vi "symmetry property.vi"() -> ()   [LabVIEW 2014]
panel:
  out "Waveform Chart":dbl[][](graph)
  out "Waveform Chart 2":dbl[][](graph)
  out "OUTPUT 2":cdb[](array[numeric])
  in  "N 2":dbl
  in  "N":dbl
  in  "stop 2":bool
  out "OUTPUT-1":cdb[](array[numeric])
  in  "stop":bool
  # "SYMMETRY PROPERTY-1"
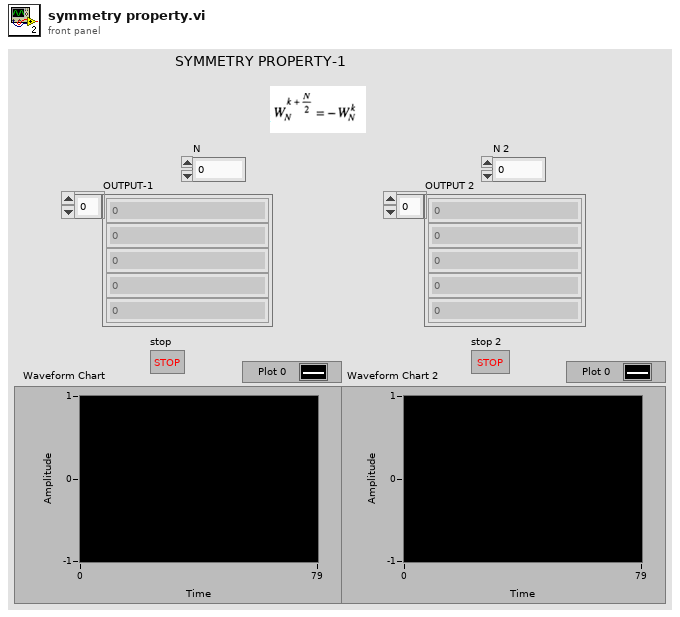
[diagram p1: front panel]
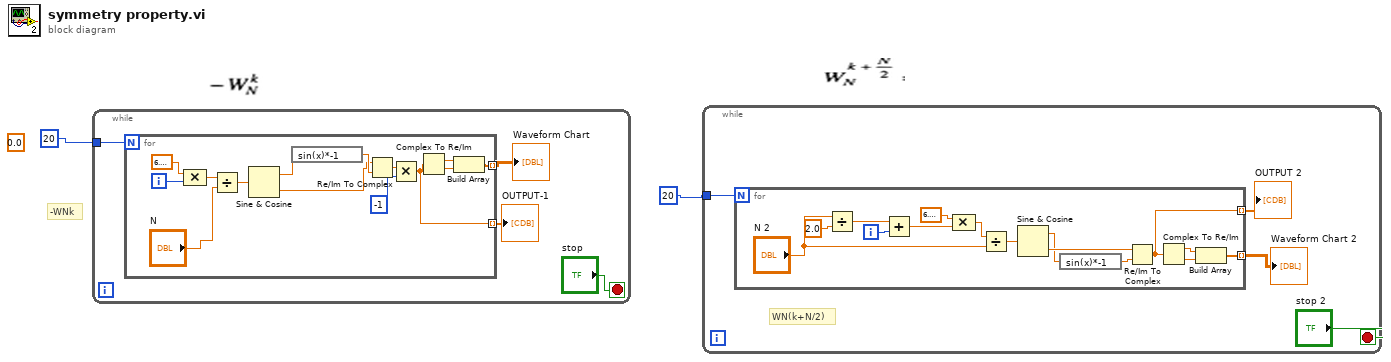
[diagram p0: block diagram]
diagram:
  (unwired) 0.0 ("Numeric")
  # "-WNk"
  n1 = while {
    tunnel: 20 -> [w6]
    stop <- "stop" stop-if-true
    n2 = for {
      N: w6 -> [_]
      tunnel: [w14] -> w3 mode=indexing
      tunnel: [w7] -> w4 mode=indexing
      i -> [w20]
      n3 = Compound Arithmetic op=MULTIPLY(6.283185307179586, w20) -> (w18:dbl)
      n4 = Divide(x=w18, y="N") -> (x/y=w17:dbl)
      n5 = Sine & Cosine(0:w17) -> (1:w11:dbl, 2:w10:dbl)
      n6 = expression code="sin(x)*-1"(w11) -> (w12:dbl)
      n7 = Re/Im To Complex(1:w12, 2:w10) -> (0:w9:cdb)
      n8 = Multiply(x=w9, y=-1) -> (x*y=w7:cdb)
      n9 = Complex To Re/Im(x + iy=w7) -> (x=w16:dbl, y=w15:dbl)
      n10 = Build Array(w16, w15) -> (w14:dbl[])
    }
    "OUTPUT-1" <- w4
    "Waveform Chart" <- w3
  }
  n11 = while {
    tunnel: 20 -> [w23]
    stop <- "stop 2" stop-if-true
    # "WN(k+N/2)"
    n12 = for {
      N: w23 -> [_]
      tunnel: [w31] -> w21 mode=indexing
      tunnel: [w25] -> w22 mode=indexing
      i -> [w29]
      n13 = Divide(x="N 2", y=2.0) -> (x/y=w27:dbl)
      n14 = Add(x=w27, y=w29) -> (x+y=w30:dbl)
      n15 = Compound Arithmetic op=MULTIPLY(6.283185307179586, w30) -> (w38:dbl)
      n16 = Divide(x=w38, y="N 2") -> (x/y=w37:dbl)
      n17 = Sine & Cosine(0:w37) -> (1:w35:dbl, 2:w36:dbl)
      n18 = expression code="sin(x)*-1"(w35) -> (w34:dbl)
      n19 = Re/Im To Complex(1:w34, 2:w36) -> (0:w25:cdb)
      n20 = Complex To Re/Im(x + iy=w25) -> (x=w33:dbl, y=w32:dbl)
      n21 = Build Array(w33, w32) -> (w31:dbl[])
    }
    "OUTPUT 2" <- w22
    "Waveform Chart 2" <- w21
  }
